vi "Write Chassis Modules.vi"(8 "error in (no error)":errorcluster, 10 "Modules":refnum<class "Module.lvclass">[](array[class]), 11 "Chassis in":refnum<class "Chassis.lvclass">) -> (0 "error out":errorcluster, 3 "Chassis out":refnum<class "Chassis.lvclass">)   [LabVIEW 2015, in "SMI.lvlib" / "Chassis.lvclass"]
uses:
  Chassis.lvclass
  Module/Module.lvclass
  Chassis.lvclass/Chassis.ctl
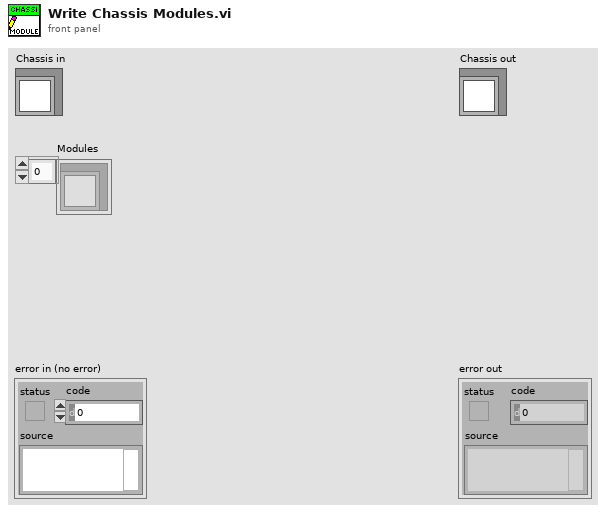
[diagram p1: front panel]
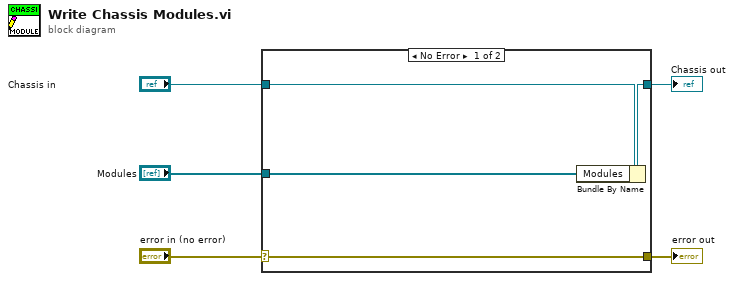
[diagram p0: block diagram]
diagram:
  n1 = case shown="No Error" "error in (no error)" {
    selector: "error in (no error)" -> [w9 w10]
    tunnel: [w9 w10] -> w4
    tunnel: [w7 w11] -> w2
    tunnel: "Chassis in" -> [w8 w11]
    tunnel: "Modules" -> [w6 _]
    frame No Error {
      n2 = Bundle By Name(cluster=w8, "Modules"=w6) -> (w7:refnum<class "Chassis.lvclass">)
    }
    frame Error {
    }
  }
  "error out" <- w4
  "Chassis out" <- w2
